vi "Ćw.1+2.vi"() -> ()   [LabVIEW 2015]
panel:
  out "<50":dbl[](array[numeric])
  out ">50":dbl[](array[numeric])
  out "Liczby":dbl[](array[numeric])
  in  "Ile liczb?":i32
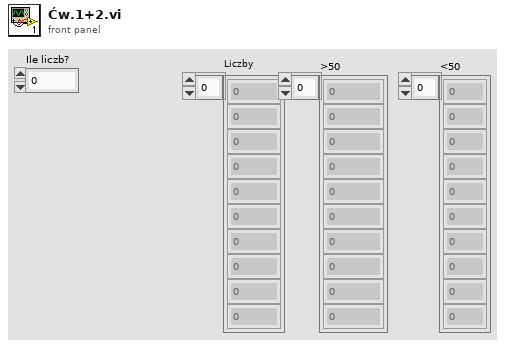
[diagram p1: front panel]
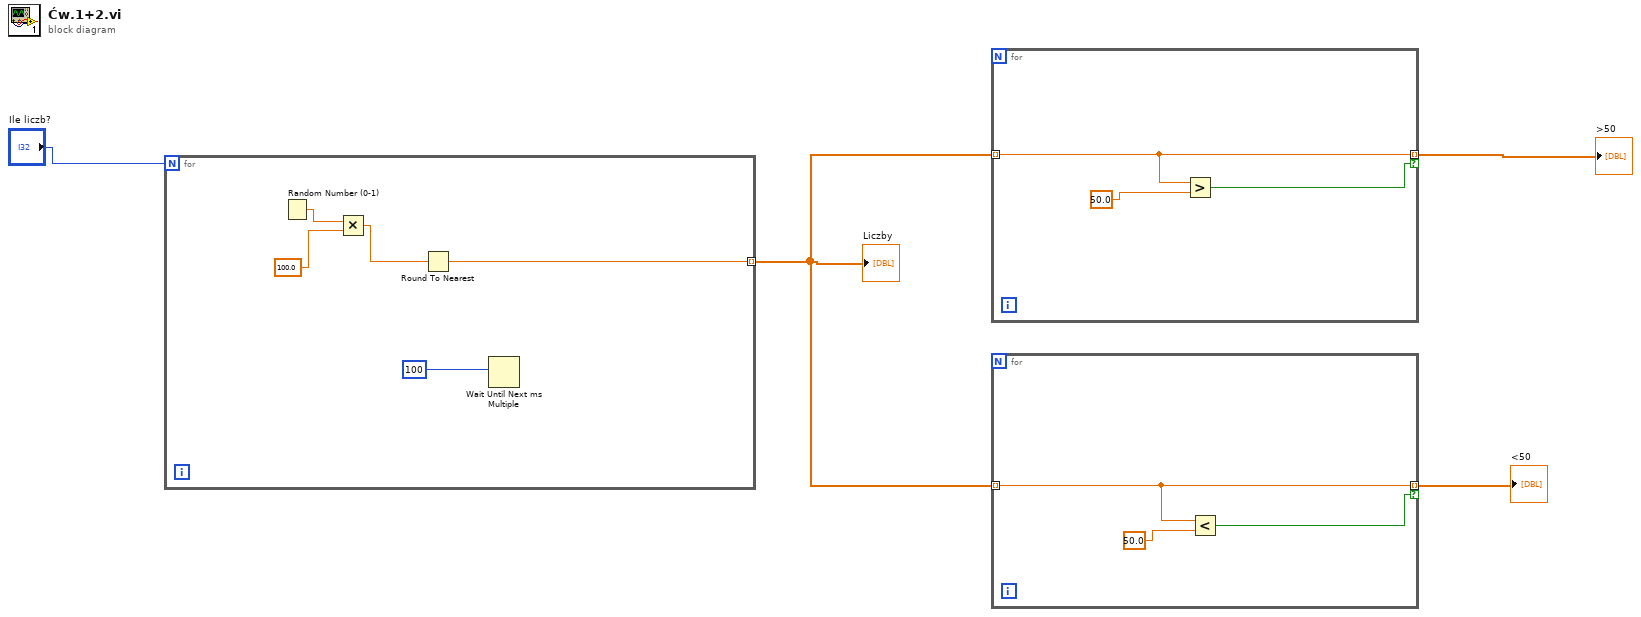
[diagram p0: block diagram]
diagram:
  n1 = for {
    N: "Ile liczb?" -> [_]
    tunnel: [w6] -> w2 mode=indexing
    n2 = Random Number (0-1)() -> (number: 0 to 1=w9:dbl)
    n3 = Multiply(x=w9, y=100.0) -> (x*y=w7:dbl)
    n4 = Round To Nearest(number=w7) -> (nearest integer value=w6:dbl)
    n5 = Wait Until Next ms Multiple(millisecond multiple=u32 100 ("millisecond timer value")) -> ()  [unwired: 1 out]
  }
  "Liczby" <- w2
  n6 = for {
    tunnel: w2 -> [w11] mode=indexing
    tunnel: [w11] -> w3 mode=indexing if=w10
    n7 = Greater?(x=w11, y=50.0) -> (0:w10:bool)
  }
  ">50" <- w3
  n8 = for {
    tunnel: [w15] -> w1 mode=indexing if=w13
    tunnel: w2 -> [w15] mode=indexing
    n9 = Less?(x=w15, y=50.0) -> (x < y?=w13:bool)
  }
  "<50" <- w1
